vi "appendChannels.vi"(8 "error in (no error)":errorcluster, 10 "ChannelArrayToAppend":refnum<class "ChannelArray.lvclass">, 11 "ChannelArray in":refnum<class "ChannelArray.lvclass">) -> (0 "error out":errorcluster, 3 "ChannelArray out":refnum<class "ChannelArray.lvclass">)   [LabVIEW 2011, in "Tools.lvlib" / "DatabaseHelpers.lvlib" / "ChannelArray.lvclass"]
uses:
  ChannelArray.lvclass
  ChannelArray.lvclass/ChannelArray.ctl
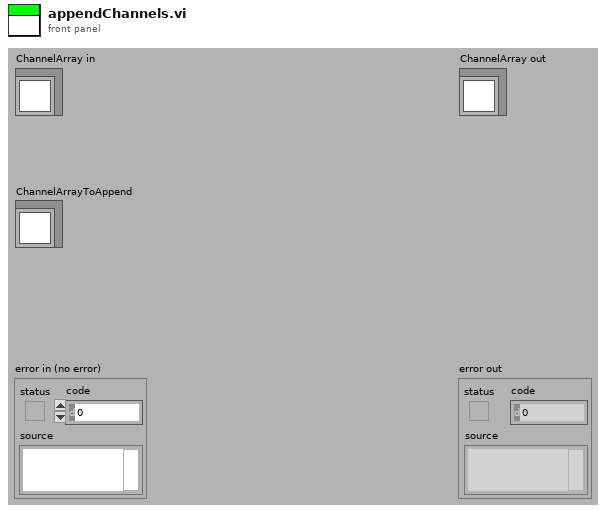
[diagram p1: front panel]
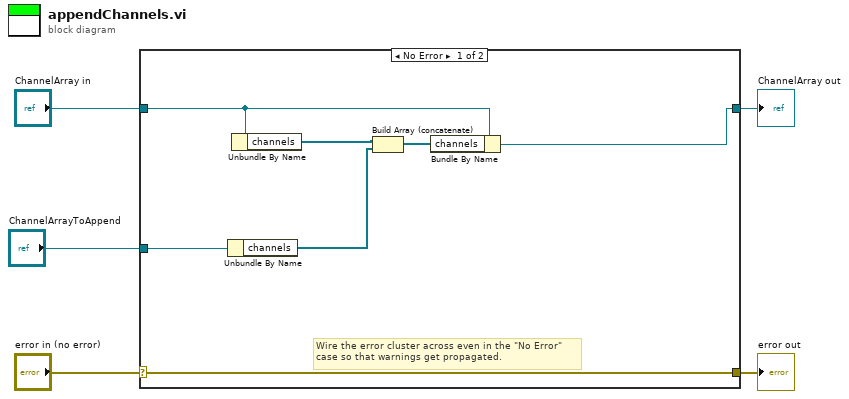
[diagram p0: block diagram]
diagram:
  n1 = case shown="No Error" "error in (no error)" {
    selector: "error in (no error)" -> [w12 w14]
    tunnel: [w12 w14] -> w4
    tunnel: [w6 w13] -> w2
    tunnel: "ChannelArray in" -> [w7 w13]
    tunnel: "ChannelArrayToAppend" -> [w11 _]
    frame No Error {
      # "Wire the error cluster across even in the \"No Error\"\ncase so that warnings get propagated."
      n2 = Unbundle By Name(w11) -> ("channels"=w9:refnum<class "Channel.lvclass">[])
      n3 = Unbundle By Name(w7) -> ("channels"=w10:refnum<class "Channel.lvclass">[])
      n4 = Build Array (concatenate)(w10, w9) -> (w8:refnum<class "Channel.lvclass">[])
      n5 = Bundle By Name(cluster=w7, "channels"=w8) -> (w6:refnum<class "ChannelArray.lvclass">)
    }
    frame Error {
    }
  }
  "error out" <- w4
  "ChannelArray out" <- w2
